vi "PowI64.vi"(4 "y":i64, 5 "x":i64) -> (1 "x^y":i64, 2 "Overflow?":bool)   [LabVIEW 2017, in "GPOverflow.lvlib"]
doc: "Computes <B>x</B> to the <B>y</B>'th power keeping track of numeric overflow.\n\n<B>Overflow?</B> will be True if positive or negative overflow occurred. The output will saturate in case of overflow.\n\nThis VI is inlined.\n\nSteen Schmidt\nGPower\n8/8 2013"
uses:
  GPOverflow.lvlib
  Mult/MultI64.vi
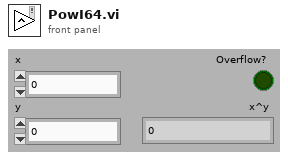
[diagram p1: front panel]
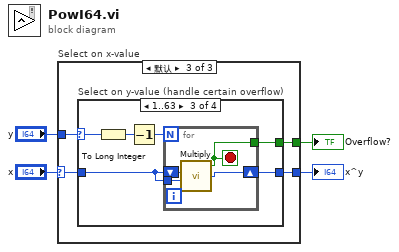
[diagram p0: block diagram]
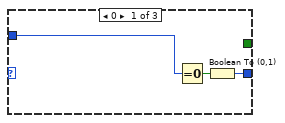
[diagram p2: hidden frame]
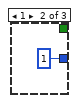
[diagram p3: hidden frame]
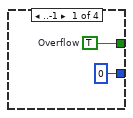
[diagram p4: hidden frame]
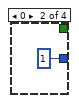
[diagram p5: hidden frame]
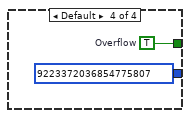
[diagram p6: hidden frame]
diagram:
  n1 = case "Select on x-value" shown="默认" "x" {
    selector: "x" -> [_ _ w10]
    tunnel: [_ _ w12] -> w4
    tunnel: [w5 i64 1 ("x") w11] -> w3
    tunnel: "y" -> [w7 _ w9]
    frame 0 {
      n2 = Equal To 0?(x=w7) -> (x = 0?=w6:bool)
      n3 = Boolean To (0,1)(Boolean=w6) -> (0, 1=w5:i16)
    }
    frame 1 {
    }
    frame Default {
      n4 = case "Select on y-value (handle certain overflow)" shown="1..63" w9 {
        selector: w9 -> [_ _ w16 _]
        tunnel: [w14 _ w19 w27] -> w12
        tunnel: [i64 0 ("x") i64 1 ("x") w18 i64 9223372036854775807 ("x")] -> w11
        tunnel: w10 -> [_ _ w17 _]
        frame ..-1 {
          w14 = TRUE  # Overflow
        }
        frame 0 {
        }
        frame 1..63 {
          n5 = To Long Integer(number=w16) -> (32bit integer=w21:i32)
          n6 = Decrement(x=w21) -> (x-1=w20:i32)
          n7 = for {
            N: w20 -> [_]
            shift-right: [w23] -> w18
            shift-left: w17 -> [w25]
            tunnel: w17 -> [w24]
            tunnel: [w22] -> w19
            stop <- w22 stop-if-true
            n8 = call-poly "Multiply.vi"("y"=w24, "x"=w25) -> ("x*y"=w23:i64, "Overflow?"=w22:bool)  [unwired: 3 in]
          }
        }
        frame Default {
          w27 = TRUE  # Overflow
        }
      }
    }
  }
  "x^y" <- w3
  "Overflow?" <- w4
